vi "NewConcreteCreatorB.vi"(8 "error in (no error)":errorcluster) -> (0 "error out":errorcluster, 3 "ConcreteCreatorA out":refnum<class "ConcreteCreatorB.lvclass">)   [LabVIEW 2020, in "FactoryMethod.lvlib" / "ConcreteCreatorB.lvclass"]
uses:
  ConcreteCreatorB.lvclass
  ConcreteCreatorB.lvclass/ConcreteCreatorB.ctl
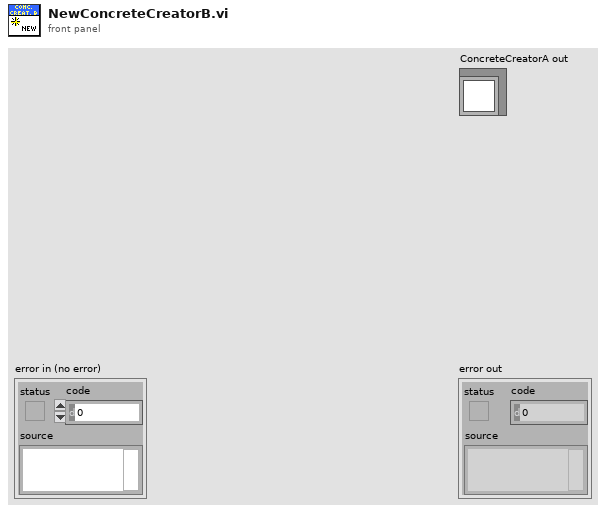
[diagram p1: front panel]
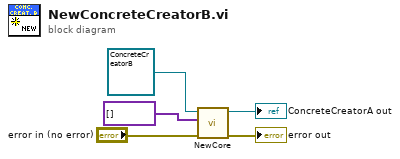
[diagram p0: block diagram]
diagram:
  n1 = call-dynamic "NewCore.vi"("error in (no error)"="error in (no error)", "ParamsArray"=variant[] [], "ConcreteCreatorA in"=refnum<class "ConcreteCreatorB.lvclass"> refnum) -> ("error out"=→"error out":errorcluster, "ConcreteCreatorA out"=→"ConcreteCreatorA out":refnum<class "ConcreteCreatorB.lvclass">)  [unwired: 7 in]
